vi "Example (single).vi"() -> ()   [LabVIEW 2017]
uses:
  Example.ctl
  source/TreeLUT.lvclass
panel:
  out "Attribute":string
  in  "Stop":bool
  out "Value":variant
  in  "CTD Tree":string(tree)
  in  "Example":T1={"Numeric"={"I32"=0, "DBL"=0.0}, "Boolean"={"Boolean"=TRUE}, "String"={"String"="", "Path"=path ""}, "Timing"={"Time Stamp"=timestamp(0 s since 1904-01-01), "Waveform"={"t0"=timestamp(0 s since 1904-01-01), "dt"=1.0, "Y"=[]}}, "Objects & Variants"={"LabVIEW Object"=refnum, "Variant"=variant}, "Refnum"={"NAR"=refnum, "DigNum"=refnum, "queue"=refnum, "notifier"=refnum}}
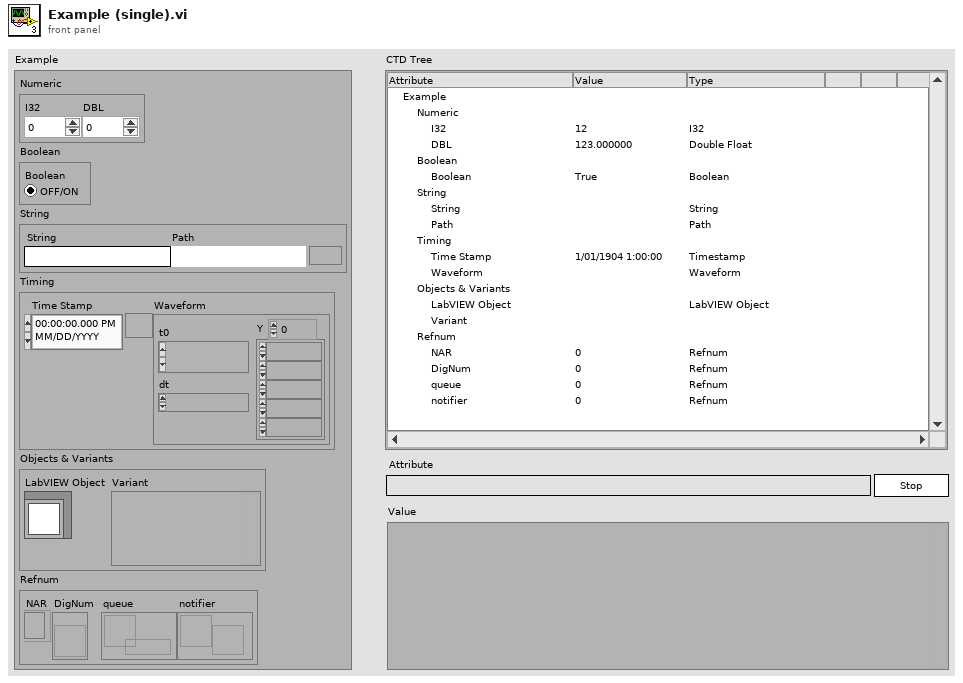
[diagram p1: front panel]
types:
  T1 = typedef "Example.ctl" = cluster{"Numeric":cluster{"I32":i32, "DBL":dbl}, "Boolean":cluster{"Boolean":bool}, "String":cluster{"String":string, "Path":path}, "Timing":cluster{"Time Stamp":timestamp, "Waveform":waveform(dbl)}, "Objects & Variants":cluster{"LabVIEW Object":refnum<class>, "Variant":variant}, "Refnum":cluster{"NAR":refnum<file>, "DigNum":refnum<vi>, "queue":refnum<queue>, "notifier":refnum<notifier>}}
  T2 = cluster{"Left Cell String":string, "Child Text":string[], "Child Tag":string, "Item Indent":i32, "Child Only?":bool, "Glyph Index":i32}[]
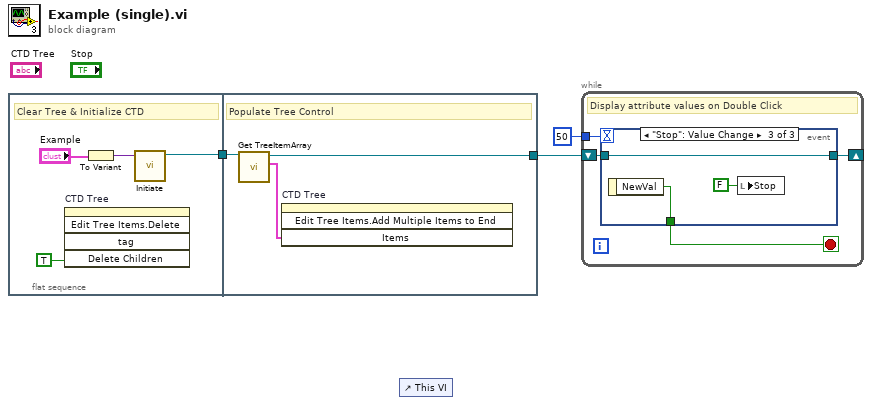
[diagram p0: block diagram]
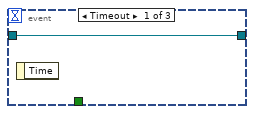
[diagram p2: hidden frame]
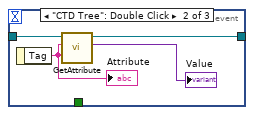
[diagram p3: hidden frame]
diagram:
  n1 = flat-sequence {
    tunnel: [w4] -> w3
    tunnel: w3 -> [w9]
    tunnel: [w8] -> w2
    frame #0 {
      # "Clear Tree & Initialize CTD"
      n2 = invoke on="CTD Tree" class="Tree (strict)" method="Edit Tree Items.Delete"("Delete Children"=TRUE) -> ()  [unwired: 4 in, 5 out]
      n3 = To Variant(anything="Example") -> (Variant=w5:variant)
      n4 = call "Initiate.vi"("Raw Variant"=w5) -> ("ClusterTree out"=w4:refnum<class "TreeLUT.lvclass">)  [unwired: 9 in, 1 out]
    }
    frame #1 {
      # "Populate Tree Control"
      n5 = call "Get TreeItemArray.vi"("ClusterTree in"=w9) -> ("TreeItem Array"=w10:T2, "ClusterTree out"=w8:refnum<class "TreeLUT.lvclass">)  [unwired: 8 in, 1 out]
      n6 = invoke on="CTD Tree" class="Tree (strict)" method="Edit Tree Items.Add Multiple Items to End"("Items"=w10) -> ()  [unwired: 3 in, 4 out]
    }
  }
  n7 = control-ref of="This VI"() -> ()  [unwired: 1 out]
  n8 = while {
    shift-right: [w13] -> _
    shift-left: w2 -> [w14]
    tunnel: 50 -> [w12]
    stop <- w11 stop-if-true
    # "Display attribute values on Double Click"
    n9 = event shown="[2] \"Stop\": Value Change" {
      selector: _ -> [_ _ _]
      dyn-events: _ -> [_ _ _]
      timeout: w12 -> [_ _ _]
      tunnel: w14 -> [w15 w18 w21]
      tunnel: [w15 w17 w21] -> w13
      tunnel: [_ _ w22] -> w11
      event Timeout {
        n10 = event-data() -> ()  [unwired: 1 in, 1 out]
      }
      event "CTD Tree": Double Click {
        n11 = event-data() -> ("Tag"=w16:string)  [unwired: 1 in]
        "Attribute" <- w16
        n12 = call "GetAttribute.vi"("Attribute"=w16, "ClusterTreeDict in"=w18) -> ("Value"=→"Value":variant, "ClusterTreeDict out"=w17:refnum<class "TreeLUT.lvclass">)  [unwired: 7 in, 1 out]
      }
      event "Stop": Value Change {
        n13 = event-data() -> ("NewVal"=w22:bool)  [unwired: 1 in]
        n14 = local write "Stop"(FALSE ("Stop")) -> ()
      }
    }
  }
